vi "FindAllLVDepsSubVIs.vi"(8 "error in (no error)":errorcluster, 11 "Project Path":path=path "E:/sw-deps-monitor/Source/BuildSpecs/Modules/ModuleA.lvproj") -> (0 "error out":errorcluster, 2 "Descendents SubVIsQualified Name":string[][](array[string]), 3 "LV Descendents Qualified Name":string[](array[string]))   [LabVIEW 2019, in "Hawkeye.lvlib"]
uses:
  Hawkeye.lvlib
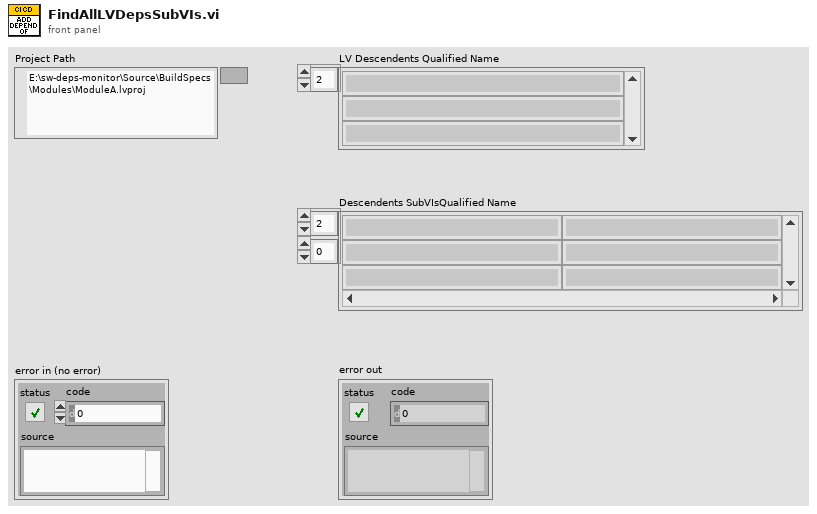
[diagram p1: front panel]
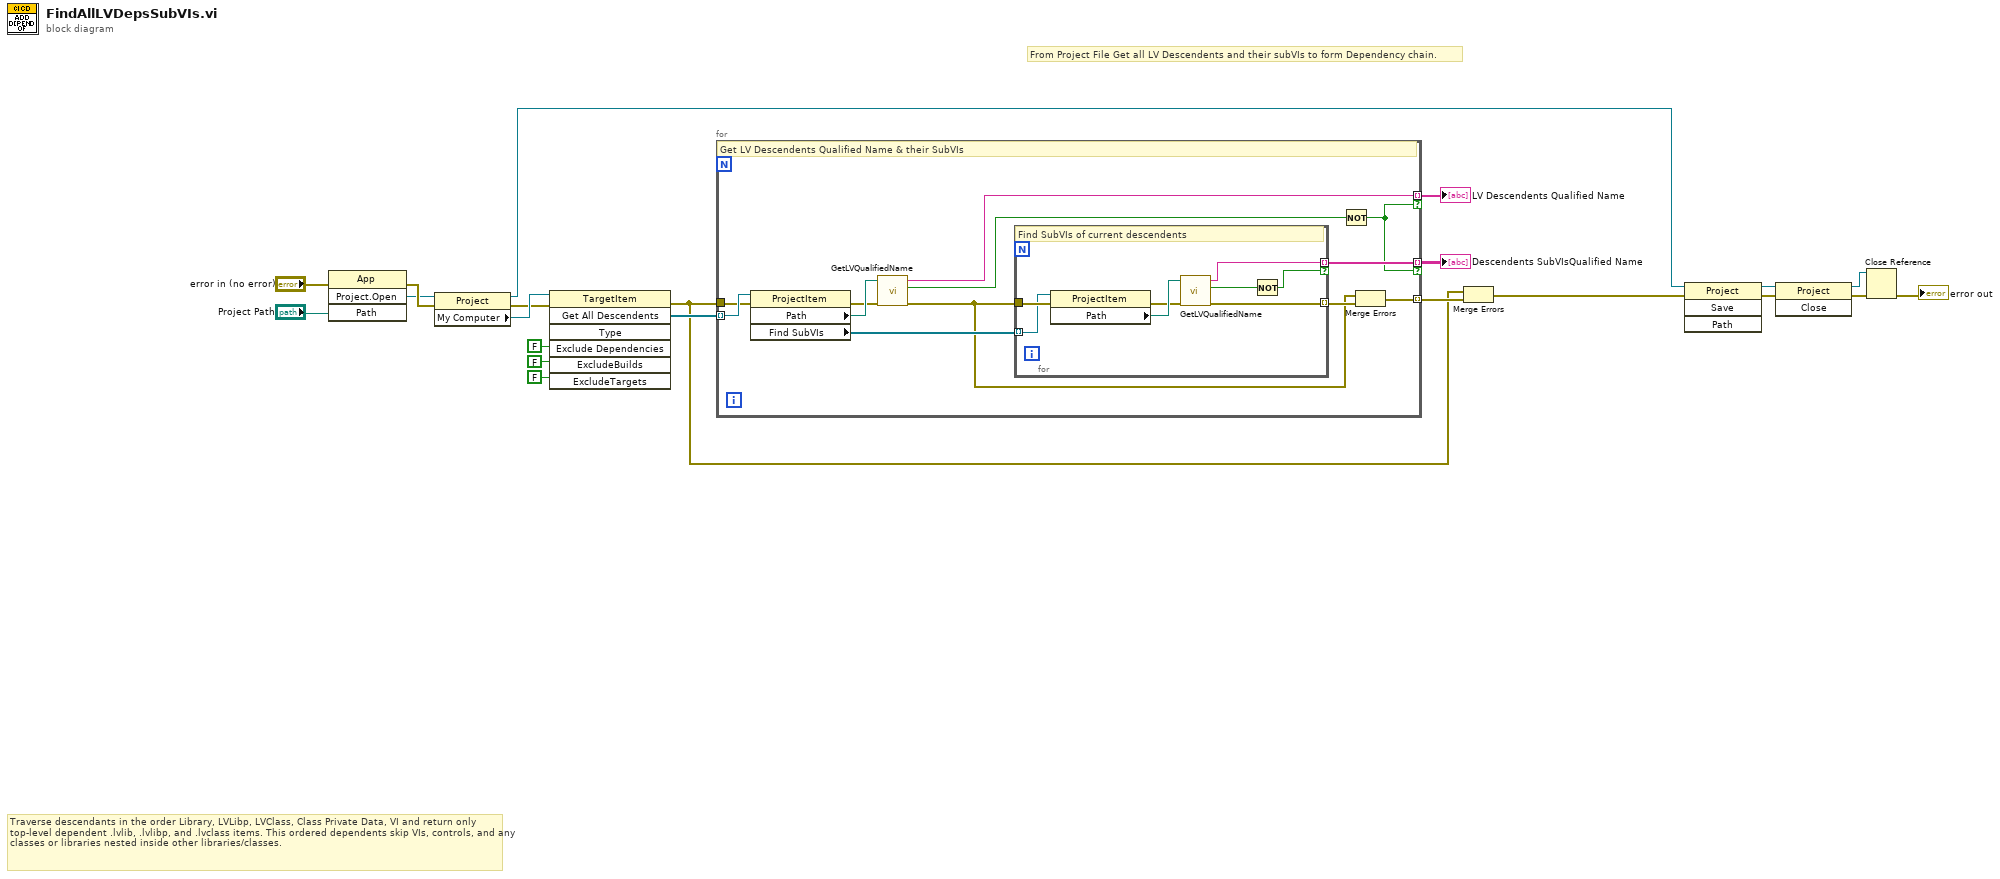
[diagram p0: block diagram]
diagram:
  # "From Project File Get all LV Descendents and their subVIs to form Dependency chain."
  # "Traverse descendants in the order Library, LVLibp, LVClass, Class Private Data, VI and return only top-level dependent .lvlib, .lvlibp, and .lvclass items. This ordered dependents skip VIs, controls, and any classes or libraries nested inside other libraries/classes."
  n1 = invoke class="App" method="Project.Open"(error in="error in (no error)", "Path"="Project Path") -> (error out=w20:errorcluster, "Project:Open"=w19:refnum<vi>)  [unwired: 2 in, 2 out]
  n2 = property class="Project"(reference=w19, error in=w20) -> (reference out=w12:refnum<vi>, error out=w14:errorcluster, "My Computer"=w15:refnum<vi>)
  n3 = invoke class="TargetItem" method="Get All Descendents"(reference=w15, error in=w14, "Exclude Dependencies"=FALSE ("ExcludeDependencies"), "ExcludeBuilds"=FALSE, "ExcludeTargets"=FALSE) -> (error out=w1:errorcluster, "All Descendents"=w3:refnum<vi>[])  [unwired: 2 in, 5 out]
  n4 = for {
    tunnel: w3 -> [w33] mode=indexing
    tunnel: [w30] -> w5 mode=indexing if=w28
    tunnel: [w27] -> w4 mode=indexing if=w28
    tunnel: w1 -> [w26]
    tunnel: [w23] -> w2 mode=indexing
    # "Get LV Descendents Qualified Name & their SubVIs"
    n5 = property class="ProjectItem"(reference=w33, error in=w26) -> (error out=w24:errorcluster, "Path"=w25:path, "Find SubVIs"=w31:refnum<vi>[])  [unwired: 1 out]
    n6 = call "GetLVQualifiedName.vi"("error in (no error)"=w24, "LV File Path"=w25) -> ("error out"=w22:errorcluster, "Non LabVIEW File?"=w29:bool, "VI Name / CTL Name / LVCLASS Name"=w27:string)  [unwired: 7 in]
    n7 = for {
      tunnel: w31 -> [w40] mode=indexing
      tunnel: [w38] -> w30 mode=indexing if=w36
      tunnel: w22 -> [w41]
      tunnel: [w34] -> w32 mode=indexing
      # "Find SubVIs of current descendents"
      n8 = property class="ProjectItem"(reference=w40, error in=w41) -> (error out=w35:errorcluster, "Path"=w39:path)  [unwired: 1 out]
      n9 = call "GetLVQualifiedName.vi"("error in (no error)"=w35, "LV File Path"=w39) -> ("error out"=w34:errorcluster, "Non LabVIEW File?"=w37:bool, "VI Name / CTL Name / LVCLASS Name"=w38:string)  [unwired: 7 in]
      n10 = Not(x=w37) -> (.not. x?=w36:bool)
    }
    n11 = Not(x=w29) -> (.not. x?=w28:bool)
    n12 = Merge Errors(w22, w32) -> (w23:errorcluster)
  }
  "Descendents SubVIsQualified Name" <- w5
  "LV Descendents Qualified Name" <- w4
  n13 = Merge Errors(w1, w2) -> (w13:errorcluster)
  n14 = invoke class="Project" method="Save"(reference=w12, error in=w13) -> (reference out=w9:refnum<vi>, error out=w7:errorcluster)  [unwired: 2 in, 2 out]
  n15 = invoke class="Project" method="Close"(reference=w9, error in=w7) -> (reference out=w8:refnum<vi>, error out=w6:errorcluster)  [unwired: 1 in, 1 out]
  n16 = Close Reference(reference=w8, error in (no error)=w6) -> (error out=→"error out":errorcluster)
